vi "2B_Tech Serial Data Recording & DECADE 2.0(serial_sim).vi"() -> ()   [LabVIEW 2014]
uses:
  <vilib>/Platform/TimedLoop/XDataNode/timing_clust.ctl
  <vilib>/Platform/TimedLoop/XDataNode/nitl_modes.ctl
  <vilib>/Platform/TimedLoop/XDataNode/wakeup.ctl
  <vilib>/Utility/error.llb/whitespace.ctl
  <vilib>/Utility/tcp.llb/UDP Multicast Read-Only Open.vi
  <vilib>/Utility/tcp.llb/UDP Multicast Write-Only Open.vi
  <vilib>/platform/TimedLoop/XDataNode/XDataNode.xnode
  <vilib>/Platform/TimedLoop/XDataNode/XDNodeRunTimeDep.lvlib
  <vilib>/Instr/_visa.llb/VISA Configure Serial Port (Instr).vi
  <vilib>/Instr/_visa.llb/VISA Flush IO Buffer Mask.ctl
  <vilib>/Instr/_visa.llb/VISA Set IO Buffer Mask.ctl
panel:
  in  "timeout (10sec)":u32=3000
  in  "VISA resource name":refnum<visa-resource-name>="ASRL2::INSTR"
  in  "Ambient or Cabin Mode":bool
  in  "Simulate 3 av":dbl
  in  "Simulate\nConc":i32
  in  "Simulate\nconc":bool
  in  "3hr_alm_thresh":i32=80
  out "3hrAvg_Alarm":bool
  out "Inst_Alarm":bool
  in  "Inst_alm_thresh":i32=220
  out "Time":string
  in  "Clear Display\nErrors":bool
  out "Read Error Counter\nfrom process loop":u32
  out "CABOZO UDP_ASCII_Out":string
  out "Ozo_array":string[](array[string])
  out "3hr_ozo_avg":dbl
  out "q_size":i32
  out "Data Output":string[](array[string])
  out "UDP packet\nSend status":bool
  out "TWBOZO UDP_ASCII_Out":string
  in  "spare_2":string="0"
  in  "spare_1":string="0"
  out "UDP_Out_Error":errorcluster
  out "UDP_Pack_num":u32
  out "UDP_In_Error":errorcluster
  out "UDP_In":string
  in  "Flight Number":string
  out "Number of times \nRead time out":u32
  out "Data Loop count":i32
  out "2B_Serial_error out":errorcluster
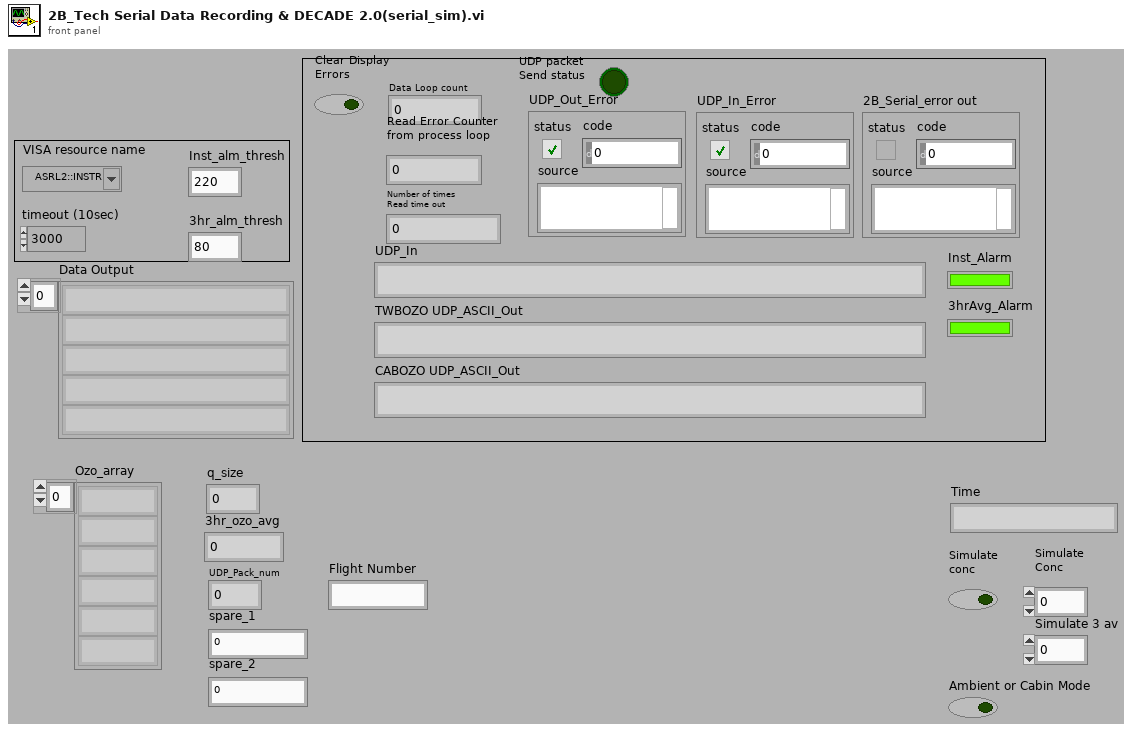
[diagram p1: front panel]
types:
  T1 = typedef "VISA Flush IO Buffer Mask.ctl" = u16
  T2 = typedef "VISA Set IO Buffer Mask.ctl" = u16
  T3 = typedef "XDNodeRunTimeDep.lvlib/timing_clust.ctl" = cluster{"Expected End [f-1]":u64, "Actual End [f-1]":u64, "Finished Late? [f-1]":bool, "Expected End [i-1]":u64, "Actual End [i-1]":u64, "Finished Late? [i-1]":bool, "Expected Start [i]":u64, "Actual Start [i]":u64, "Expected Start [f]":u64, "Actual Start [f]":u64, "Source Name":string, "Structure Name":string, "Period":i64, "Deadline":i64, "Offset":i64, "Start":i64, "Priority":i32, "Timeout":i32, "Mode":T4, "Wakeup Reason":T5, "Error":errorcluster, "Source Type":string, "Secondary Source Type":string, "Global End Time":u64, "Global Start Time":u64, "Frame Duration":u64, "Iteration Duration":u64, "Assigned CPU":i32, "I/O Scan Engine Mode":u32}
  T4 = typedef "XDNodeRunTimeDep.lvlib/nitl_modes.ctl" = enum32{"No Change", "Process missed periods, maintain original phase", "Discard missed periods, maintain original phase", "Process missed periods, ignore original phase", "Discard missed periods, ignore original phase"}
  T5 = typedef "XDNodeRunTimeDep.lvlib/wakeup.ctl" = enum32{"Normal", "Aborted", "Asynchronous wakeup", "Timing source error", "Timed loop error", "Timeout"}
  T6 = typedef "whitespace.ctl" = u16
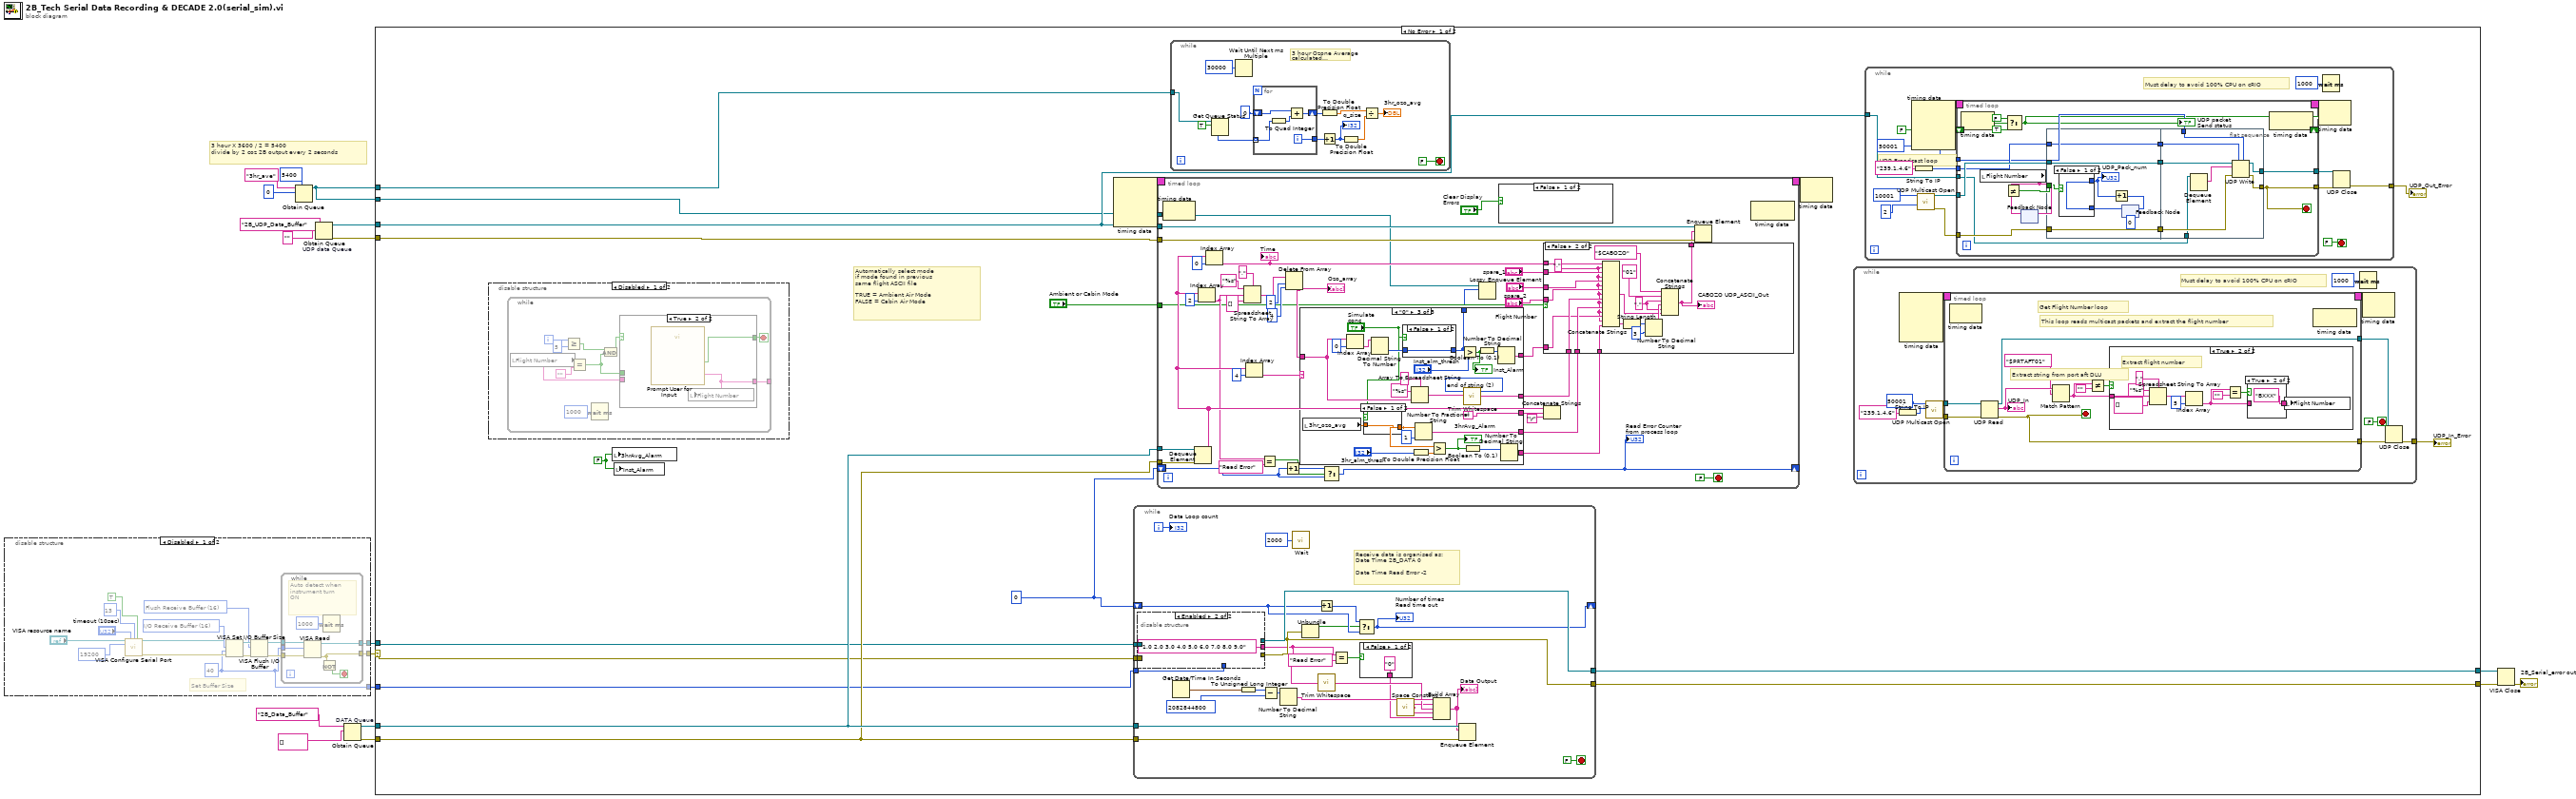
[diagram p0: block diagram]
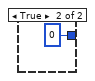
[diagram p5: hidden frame]
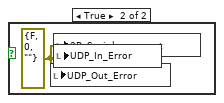
[diagram p6: hidden frame]
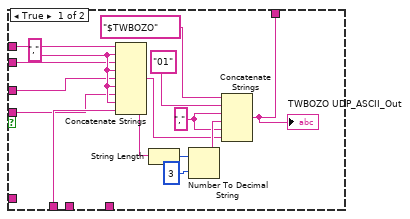
[diagram p7: hidden frame]
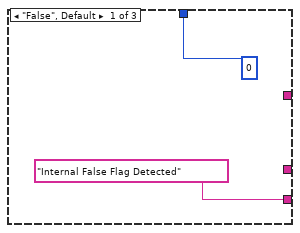
[diagram p8: hidden frame]
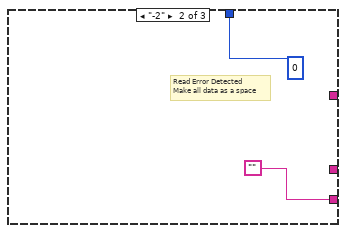
[diagram p9: hidden frame]
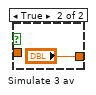
[diagram p10: hidden frame]
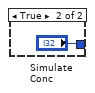
[diagram p11: hidden frame]
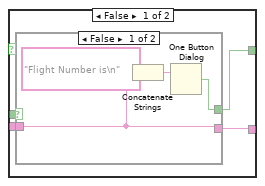
[diagram p12: hidden frame]
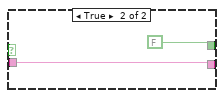
[diagram p13: hidden frame]
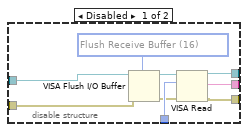
[diagram p15: hidden frame]
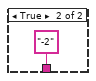
[diagram p16: hidden frame]
diagram:
  # "3 hour X 3600 / 2 = 5400\ndivide by 2 coz 2B output every 2 seconds"
  n1 = disable-structure shown="Disabled" {
    disable-tunnel: [w21 _] -> w3
    disable-tunnel: [w20 _] -> w2
    disable-tunnel: [w19 _] -> w1
    frame Disabled {
      w19 = u32 40 ("size (4096)")
      w26 = T1 16 items=["Flush Receive Buffer"=16, "Write Transmit Buffer to Device"=32, "Flush Receive Buffer (No I/O)"=64, "Flush Transmit Buffer"=128] ("Mask")
      w27 = T2 16 items=["I/O Receive Buffer"=16, "I/O Transmit Buffer"=32, "I/O Receive and Transmit Buffer"=48] ("Mask")
      # "Set Buffer Size"
      n2 = call-poly "VISA Configure Serial Port"("VISA resource name"="VISA resource name", "timeout (10sec)"="timeout (10sec)", "termination char\n(0xA = '\\n' = LF)"=u8 13 ("termination char\n(0xA = '\\n' = LF)"), "Enable Termination\nChar (T)"=TRUE ("Enable Termination\nChar (T)"), "baud rate (9600)"=u32 19200) -> ("VISA resource name out"=w25:refnum<visa-resource-name>, "error out"=w24:errorcluster)  [unwired: 9 in]
      n3 = VISA Set I/O Buffer Size(VISA resource name=w25, mask (16)=w27, size (4096)=w19, error in (no error)=w24) -> (VISA resource name out=w28:refnum<visa-resource-name>, error out=w29:errorcluster)
      n4 = VISA Flush I/O Buffer(VISA resource name=w28, mask (16)=w26, error in (no error)=w29) -> (VISA resource name out=w23:refnum<visa-resource-name>, error out=w22:errorcluster)
      n5 = while {
        tunnel: w19 -> [w41]
        tunnel: w23 -> [w40]
        tunnel: w22 -> [w39]
        tunnel: [w37] -> w21
        tunnel: [w36] -> w20
        stop <- w38 stop-if-true
        # "Auto detect when\ninstrument turn\nON"
        n6 = VISA Read(VISA resource name=w40, byte count=w41, error in (no error)=w39) -> (VISA resource name out=w36:refnum<visa-resource-name>, error out=w37:errorcluster)  [unwired: 2 out]
        n7 = Not(x=w37) -> (.not. x?=w38:bool)
        n8 = Wait (ms)(milliseconds to wait=u32 1000) -> ()  [unwired: 1 out]
      }
    }
    frame Enabled {
    }
  }
  n9 = Obtain Queue(max queue size (-1, unlimited)=5400, name (unnamed)="3hr_ave", element data type=0 ("index")) -> (queue out=w4:refnum<queue>)  [unwired: 2 in, 2 out]
  n10 = Obtain Queue "UDP data Queue"(name (unnamed)="2B_UDP_Data_Buffer", element data type="") -> (queue out=w10:refnum<queue>, error out=w9:errorcluster)  [unwired: 3 in, 1 out]
  n11 = Obtain Queue "DATA Queue"(name (unnamed)="2B_Data_Buffer", element data type=string[] []) -> (queue out=w14:refnum<queue>, error out=w13:errorcluster)  [unwired: 3 in, 1 out]
  n12 = case shown="No Error" w3 {
    selector: w3 -> [w43 w336]
    tunnel: w2 -> [w44 w337]
    tunnel: [w59 w337] -> w17
    tunnel: [w51 w336] -> w18
    tunnel: w14 -> [w58 _]
    tunnel: w13 -> [w57 _]
    tunnel: w10 -> [w55 _]
    tunnel: w9 -> [w56 _]
    tunnel: w4 -> [w54 _]
    tunnel: w4 -> [w53 _]
    tunnel: w1 -> [w42 _]
    frame No Error {
      w50 = FALSE
      w52 = u32 0
      # "Automatically select mode\nif mode found in previous\nsame flight ASCII file\n\nTRUE = Ambient Air Mode\nFALSE = Cabin Air Mode"
      n13 = disable-structure shown="Disabled" {
        frame Disabled {
          n14 = while {
            tunnel: [w282] -> _
            i -> [w281]
            stop <- w284 stop-if-true
            n15 = local read "Flight Number"() -> (w276:string)
            n16 = Greater Or Equal?(x=w281, y=5) -> (x >= y?=w279:bool)
            n17 = Equal?(x=w276, y="") -> (x = y?=w277:bool)
            n18 = Wait (ms)(milliseconds to wait=u32 1000) -> ()  [unwired: 1 out]
            n19 = And(x=w279, y=w277) -> (x .and. y?=w278:bool)
            n20 = case shown="True" w278 {
              tunnel: [w286 w297] -> w284
              tunnel: [w287 w296] -> w282
              tunnel: w277 -> [w289 _]
              tunnel: w276 -> [w288 _]
              frame False {
                n21 = case shown="False" w289 {
                  tunnel: [w291 w295] -> w287
                  tunnel: w288 -> [w291 w295]
                  tunnel: [w293 FALSE] -> w286
                  frame False {
                    n22 = Concatenate Strings("Flight Number is\n" ("string"), w291) -> (w290:string)
                    n23 = One Button Dialog(message=w290) -> (true=w293:bool)  [unwired: 1 in]
                  }
                  frame True {
                  }
                }
              }
              frame True {
                n24 = call "Prompt User for Input"() -> ("Flight Number BXXX"=w296:string, "OK"=w297:bool)  [unwired: 17 in, 1 out]
                n25 = local write "Flight Number"(w296) -> ()
              }
            }
          }
        }
        frame Enabled {
        }
      }
      n26 = local write "3hrAvg_Alarm"(w50) -> ()
      n27 = local write "Inst_Alarm"(w50) -> ()
      n28 = node-c288() -> (w49:T3)  [unwired: 4 in]
      n29 = while {
        tunnel: [w314] -> w51
        shift-right: [w320] -> _
        shift-left: w52 -> [w321]
        tunnel: [w323] -> w59
        tunnel: w44 -> [w319]
        tunnel: w43 -> [w318]
        tunnel: w58 -> [w317]
        tunnel: w57 -> [w316]
        tunnel: w42 -> [w315]
        i -> [w322]
        stop <- FALSE stop-if-true
        # "Receive data is organised as:\nDate Time 2B_DATA 0\n\nDate Time Read Error -2"
        n30 = disable-structure shown="Enabled" {
          disable-tunnel: [w332 _] -> w323
          disable-tunnel: w319 -> [w331 _]
          disable-tunnel: w318 -> [w330 _]
          disable-tunnel: w315 -> [w329 _]
          disable-tunnel: [w328 _] -> w314
          disable-tunnel: [w324 "1.0 2.0 3.0 4.0 5.0 6.0 7.0 8.0 9.0" ("string")] -> w300
          frame Disabled {
            w326 = T1 16 items=["Flush Receive Buffer"=16, "Write Transmit Buffer to Device"=32, "Flush Receive Buffer (No I/O)"=64, "Flush Transmit Buffer"=128] ("Mask")
            n31 = VISA Flush I/O Buffer(VISA resource name=w331, mask (16)=w326, error in (no error)=w330) -> (VISA resource name out=w327:refnum<visa-resource-name>, error out=w325:errorcluster)
            n32 = VISA Read(VISA resource name=w327, byte count=w329, error in (no error)=w325) -> (VISA resource name out=w332:refnum<visa-resource-name>, read buffer=w324:string, error out=w328:errorcluster)  [unwired: 1 out]
          }
          frame Enabled {
          }
        }
        n33 = Get Date/Time In Seconds() -> (seconds since 1Jan1904=w309:timestamp)
        n34 = To Unsigned Long Integer(number=w309) -> (unsigned 32bit integer=w311:u32)
        n35 = Subtract(x=w311, y=u32 2082844800) -> (x-y=w308:u32)
        n36 = Number To Decimal String(number=w308) -> (decimal integer string=w305:string)  [unwired: 1 in]
        n37 = call "Wait"("Count(mSec)"=u32 2000) -> ()  [unwired: 1 out]
        n38 = Unbundle(w314) -> ("status"=w312:bool)  [unwired: 2 out]
        n39 = Increment(x=w321) -> (x+1=w313:u32)
        n40 = call <vilib>:"Trim Whitespace.vi"("string"=w300) -> ("trimmed string"=w304:string)  [unwired: 1 in]
        n41 = Equal?(x=w300, y="Read Error") -> (x = y?=w306:bool)
        n42 = Select(t=w313, s=w312, f=w321) -> (s? t:f=w320:u32)
        "Number of times \nRead time out" <- w320
        n43 = case shown="False" w306 {
          tunnel: ["0" "-2"] -> w302
          frame False {
          }
          frame True {
          }
        }
        n44 = call <vilib>:"Space Constant.vi"() -> ("String"=w303:string)
        n45 = Build Array(w305, w303, w304, w303, w302) -> (w301:string[])
        "Data Output" <- w301
        n46 = Enqueue Element(queue=w317, element=w301, error in (no error)=w316) -> ()  [unwired: 1 in, 3 out]
        "Data Loop count" <- w322
      }
      n47 = timed-loop {
        timing: w49 -> [_]
        timing-out: [_] -> w48
        tunnel: w58 -> [w206]
        tunnel: w57 -> [w205]
        tunnel: w55 -> [w204]
        tunnel: w56 -> [w203]
        tunnel: w53 -> [w171]
        shift-right: [w176] -> _
        shift-left: w52 -> [w177]
        tunnel: "Ambient or Cabin Mode" -> [w175]
        stop <- FALSE stop-if-true
        n48 = node-c288() -> ()  [unwired: 1 in, 1 out]
        n49 = Dequeue Element(queue=w206, error in (no error)=w205) -> (element=w188:string[])  [unwired: 1 in, 3 out]
        n50 = Index Array(array=w188, index=2) -> (element=w178:string)
        n51 = Index Array(array=w188, index=0) -> (element=w190:string)
        "Time" <- w190
        n52 = Spreadsheet String To Array(delimiter (Tab)=",", format string="%s", spreadsheet string=w178, array type (2D Dbl)=string[] [] ("Values Array")) -> (array=w195:string[])
        n53 = Index Array(array=w188, index=4) -> (element=w196:string)
        n54 = Equal?(x=w178, y="Read Error") -> (x = y?=w180:bool)
        n55 = Increment(x=w177) -> (x+1=w179:u32)
        n56 = Delete From Array(array=w195, length=2, index=4) -> (array with subset deleted=w192:string[])  [unwired: 1 out]
        "Ozo_array" <- w192
        n57 = case shown="\"0\"" w196 {
          tunnel: w192 -> [_ _ w260]
          tunnel: [_ _ w263] -> w189
          tunnel: [0 0 w246] -> w170
          tunnel: ["Internal False Flag Detected" "" ""] -> w187
          tunnel: [_ _ w257] -> w182
          tunnel: [_ _ w253] -> w173
          tunnel: [_ _ w248] -> w172
          frame "False", Default {
          }
          frame "-2" {
            # "Read Error Detected\nMake all data as a space"
          }
          frame "0" {
            w264 = T6 2 items=["both", "start of string", "end of string"] ("location (both)")
            n58 = local read "3hr_ozo_avg"() -> (w244:dbl)
            n59 = Index Array(array=w260, index=0) -> (element=w261:string)
            n60 = case shown="False" "Simulate\nconc" {
              tunnel: [w268 "Simulate 3 av"] -> w243
              tunnel: w244 -> [w268 _]
              frame False {
              }
              frame True {
              }
            }
            n61 = Decimal String To Number(string=w261) -> (number=w247:i32)  [unwired: 2 in, 1 out]
            n62 = case shown="False" "Simulate\nconc" {
              tunnel: [w270 "Simulate\nConc"] -> w246
              tunnel: w247 -> [w270 _]
              frame False {
              }
              frame True {
              }
            }
            n63 = Array To Spreadsheet String(delimiter (Tab)=",", array=w260, 3:"%s" ("format string")) -> (spreadsheet string=w265:string)
            n64 = To Double Precision Float(number="3hr_alm_thresh") -> (double precision float=w250:dbl)
            n65 = Number To Fractional String(number=w243, precision (6)=i16 1) -> (F-format string=w257:string)  [unwired: 2 in]
            n66 = Greater?(x=w243, y=w250) -> (0:w251:bool)
            "3hrAvg_Alarm" <- w251
            n67 = Greater?(x=w246, y="Inst_alm_thresh") -> (0:w254:bool)
            "Inst_Alarm" <- w254
            n68 = call <vilib>:"Trim Whitespace.vi"("string"=w265, "location (both)"=w264) -> ("trimmed string"=w263:string)
            n69 = Boolean To (0,1)(Boolean=w251) -> (0, 1=w252:i16)
            n70 = Boolean To (0,1)(Boolean=w254) -> (0, 1=w255:i16)
            n71 = Number To Decimal String(number=w255) -> (decimal integer string=w253:string)  [unwired: 1 in]
            n72 = Number To Decimal String(number=w252) -> (decimal integer string=w248:string)  [unwired: 1 in]
          }
        }
        n73 = Select(t=w179, s=w180, f=w177) -> (s? t:f=w176:u32)
        "Read Error Counter\nfrom process loop" <- w176
        n74 = Lossy Enqueue Element(queue=w171, element=w170) -> ()  [unwired: 1 in, 4 out]
        n75 = case shown="False" "Clear Display\nErrors" {
          frame False {
          }
          frame True {
            w207 = errorcluster {"status"=FALSE, "code"=0, "source"=""} ("UDP Error Out")
            n76 = local write "UDP_Out_Error"(w207) -> ()
            n77 = local write "2B_Serial_error out"(w207) -> ()
            n78 = local write "UDP_In_Error"(w207) -> ()
          }
        }
        n79 = Concatenate Strings(w188, w187, "\r") -> ()  [unwired: 1 out]
        n80 = case shown="False" w175 {
          tunnel: [w213 w231] -> w202
          tunnel: w190 -> [w212 w230]
          tunnel: w189 -> [w211 w229]
          tunnel: "spare_1" -> [w210 w228]
          tunnel: "spare_2" -> [w209 w227]
          tunnel: "Flight Number" -> [w208 w226]
          tunnel: w182 -> [_ w225]
          tunnel: w173 -> [_ w224]
          tunnel: w172 -> [_ w222]
          frame True {
            w221 = ","
            w217 = ","
            n81 = Concatenate Strings(w212, w221, w210, w221, w209, w221, w208, w221, w211) -> (w216:string)
            n82 = String Length(string=w216) -> (length=w220:i32)
            n83 = Number To Decimal String(number=w220, width (-)=i16 3) -> (decimal integer string=w218:string)
            n84 = Concatenate Strings("$TWBOZO", "01", w217, w218, w217, w216) -> (w213:string)
            "TWBOZO UDP_ASCII_Out" <- w213
          }
          frame False {
            w223 = ","
            w235 = ","
            n85 = Concatenate Strings(w230, w223, w228, w223, w227, w223, w226, w223, w229, w223, w225, w223, w224, w223, w222) -> (w234:string)
            n86 = String Length(string=w234) -> (length=w238:i32)
            n87 = Number To Decimal String(number=w238, width (-)=i16 3) -> (decimal integer string=w236:string)
            n88 = Concatenate Strings("$CABOZO", "01", w235, w236, w235, w234) -> (w231:string)
            "CABOZO UDP_ASCII_Out" <- w231
          }
        }
        n89 = Enqueue Element(queue=w204, element=w202, error in (no error)=w203) -> ()  [unwired: 1 in, 3 out]
        n90 = node-c288() -> ()  [unwired: 1 in, 1 out]
      }
      n91 = while {
        tunnel: w54 -> [w64]
        stop <- FALSE stop-if-true
        # "3 hour Ozone Average calculated\nevery 30 seconds"
        n92 = Get Queue Status(queue=w64, return elements? (F)=TRUE) -> (elements=w61:i32[])  [unwired: 1 in, 7 out]
        n93 = Wait Until Next ms Multiple(millisecond multiple=u32 30000) -> ()  [unwired: 1 out]
        n94 = for {
          tunnel: [w76] -> w71
          shift-right: [w75] -> w69
          shift-left: i64 0 -> [w74]
          tunnel: w61 -> [w72] mode=indexing
          i -> [w76]
          n95 = To Quad Integer(1:w72) -> (0:w73:i64)
          n96 = Add(x=w74, y=w73) -> (x+y=w75:i64)
        }
        n97 = Increment(x=w71) -> (x+1=w65:i32)
        "q_size" <- w65
        n98 = To Double Precision Float(number=w69) -> (double precision float=w67:dbl)
        n99 = To Double Precision Float(number=w65) -> (double precision float=w68:dbl)
        n100 = Divide(x=w67, y=w68) -> (x/y=→"3hr_ozo_avg":dbl)
      }
      n101 = node-c288(w48) -> ()  [unwired: 1 out]
      n102 = while {
        tunnel: [w79] -> w45
        stop <- FALSE stop-if-true
        # "Must delay to avoid 100% CPU on cRIO"
        n103 = node-c288() -> (w81:T3)  [unwired: 4 in]
        n104 = String To IP(1:"239.1.4.6" ("name")) -> (0:w88:u32)
        n105 = call-poly <vilib>:"UDP Multicast Open.vi"("multicast addr"=w88, "port"=u16 50001) -> ("error out"=w84:errorcluster, "connection ID"=w85:refnum<k16>)  [unwired: 7 in, 1 out]
        n106 = timed-loop {
          tunnel: w85 -> [w97]
          tunnel: w84 -> [w96]
          tunnel: [w91] -> w83
          tunnel: [w89] -> w82
          timing: w81 -> [_]
          timing-out: [_] -> w80
          stop <- w89 stop-if-true
          # "Extract string from port aft DLU"
          # "Get Flight Number loop"
          # "This loop reads multicast packets and extract the flight number"
          n107 = node-c288() -> ()  [unwired: 1 in, 1 out]
          n108 = UDP Read(connection ID=w97, 8:w96) -> (data out=w92:string, error out=w89:errorcluster, 3:w91:refnum<k16>)  [unwired: 2 in, 2 out]
          "UDP_In" <- w92
          n109 = Match Pattern(string=w92, regular expression="$PRTAFT01") -> (after substring=w93:string)  [unwired: 1 in, 3 out]
          n110 = Not Equal?(x=w93, y="") -> (x != y?=w94:bool)
          n111 = case shown="True" w94 {
            tunnel: w93 -> [_ w104]
            frame False {
            }
            frame True {
              # "Extract flight number"
              n112 = Spreadsheet String To Array(delimiter (Tab)=",", format string="%s", spreadsheet string=w104, array type (2D Dbl)=string[] []) -> (array=w106:string[])
              n113 = Index Array(array=w106, index=5) -> (element=w101:string)
              n114 = Equal?(x=w101, y="") -> (x = y?=w103:bool)
              n115 = case shown="True" w103 {
                tunnel: [w110 "BXXX"] -> w100
                tunnel: w101 -> [w110 _]
                frame False {
                }
                frame True {
                }
              }
              n116 = local write "Flight Number"(w100) -> ()
            }
          }
          n117 = node-c288() -> ()  [unwired: 1 in, 1 out]
        }
        n118 = Wait (ms)(milliseconds to wait=u32 1000) -> ()  [unwired: 1 out]
        n119 = node-c288(w80) -> ()  [unwired: 1 out]
        n120 = UDP Close(connection ID=w83, 8:w82) -> (error out=w79:errorcluster)  [unwired: 1 out]
      }
      "UDP_In_Error" <- w45
      n121 = while {
        tunnel: w55 -> [w117]
        tunnel: [w116] -> w46
        stop <- FALSE stop-if-true
        # "Must delay to avoid 100% CPU on cRIO"
        # "UDP Broadcast loop"
        n122 = node-c288() -> (w119:T3)  [unwired: 4 in]
        n123 = String To IP(1:"239.1.4.6" ("name")) -> (0:w121:u32)
        n124 = call-poly <vilib>:"UDP Multicast Open.vi"("time-to-live (1)"=u16 2, "port"=u16 10001) -> ("error out"=w128:errorcluster, "connection ID"=w129:refnum<k16>)  [unwired: 8 in]
        n125 = timed-loop {
          tunnel: w129 -> [w146]
          tunnel: w128 -> [w145]
          tunnel: [w134] -> w124
          shift-right: [w131] -> _
          shift-left: FALSE -> [w139]
          tunnel: [w130] -> w123
          tunnel: w121 -> [w136]
          tunnel: u16 50001 ("port or service name") -> [w135]
          timing: w119 -> [_]
          timing-out: [_] -> w118
          tunnel: w117 -> [w132]
          stop <- w130 stop-if-true
          n126 = node-c288() -> ()  [unwired: 1 in, 1 out]
          n127 = local read "Flight Number"() -> (w133:string)
          n128 = Select(t=FALSE, s=w139, f=TRUE) -> (s? t:f=w131:bool)
          "UDP packet\nSend status" <- w131
          n129 = feedback-in #1(w133) -> ()
          n130 = feedback #1() -> (w141:string)  [unwired: 1 in]
          n131 = Not Equal?(x=w133, y=w141) -> (x != y?=w140:bool)
          n132 = flat-sequence {
            tunnel: w136 -> [w154]
            tunnel: w145 -> [w155]
            tunnel: w146 -> [w156]
            tunnel: [w156] -> w144
            tunnel: [w155] -> w143
            tunnel: [w154] -> w142
            tunnel: w140 -> [w153]
            tunnel: w135 -> [w166]
            tunnel: w144 -> [w165]
            tunnel: w143 -> [w164]
            tunnel: w142 -> [w163]
            tunnel: [w162] -> w134
            tunnel: [w161] -> w130
            tunnel: w132 -> [w159]
            frame #0 {
              n133 = feedback #2(u32 0) -> (w150:u32)
              n134 = case shown="False" w153 {
                tunnel: w150 -> [w157 _]
                tunnel: [w157 u32 0] -> w149
                frame False {
                }
                frame True {
                }
              }
              "UDP_Pack_num" <- w149
              n135 = Increment(x=w149) -> (x+1=w151:u32)
              n136 = feedback-in #2(w151) -> ()
            }
            frame #1 {
              n137 = Dequeue Element(queue=w159) -> (element=w160:string)  [unwired: 2 in, 3 out]
              n138 = UDP Write(address=w163, port or service name=w166, connection ID=w165, data in=w160, 8:w164) -> (error out=w161:errorcluster, 3:w162:refnum<k16>)  [unwired: 1 in]
            }
          }
          n139 = node-c288() -> ()  [unwired: 1 in, 1 out]
        }
        n140 = node-c288(w118) -> ()  [unwired: 1 out]
        n141 = Wait (ms)(milliseconds to wait=u32 1000) -> ()  [unwired: 1 out]
        n142 = UDP Close(connection ID=w124, 8:w123) -> (error out=w116:errorcluster)  [unwired: 1 out]
      }
      "UDP_Out_Error" <- w46
    }
    frame Error {
    }
  }
  n143 = VISA Close(VISA resource name=w17, error in (no error)=w18) -> (error out=→"2B_Serial_error out":errorcluster)
